vi "Align Image Stacks.vi"(8 "error in (no error)":errorcluster, 10 "Transmitted Light Stack":T1[](array[typedef]), 11 "Reflected Light Stack":T1[](array[typedef])) -> (0 "error out":errorcluster, 3 "Offset":cluster{"dx":i32, "dy":i32})   [LabVIEW 2013]
uses:
  <vilib>/vision/Image Controls.llb/IMAQ Image.ctl
  <vilib>/vision/NI_Vision_Development_Module.lvlib
panel:
  # "The \"Offset\" is the displacement necessary\nto align the reflected light stack with\nthe transmitted light stack. Shift the \nreflected light stack, not the transmitted!"
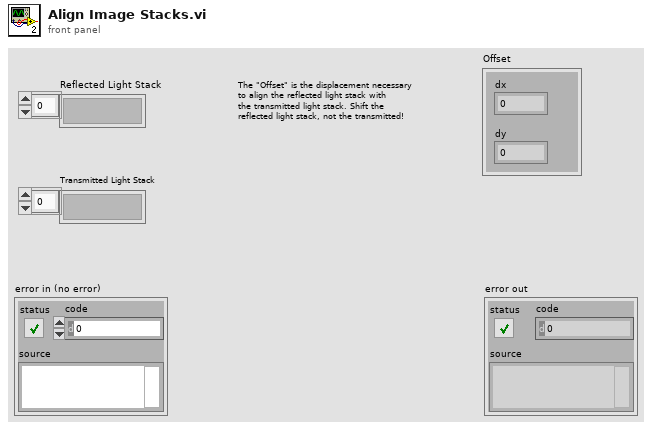
[diagram p1: front panel]
types:
  T1 = typedef "IMAQ Image.ctl" = refnum<image>
  T2 = cluster{"Number of Matches Requested":i32, "Minimum Match Score":sgl, "Angle Ranges":cluster{"Start Angle":sgl, "End Angle":sgl}[]}
  T3 = cluster{"Position":cluster{"X":sgl, "Y":sgl}, "Orientation":dbl, "Major Radius":dbl, "Minor Radius":dbl, "Score":dbl}[]
  T4 = cluster{"Position":cluster{"x":sgl, "y":sgl}, "Angle":sgl, "Scale":sgl, "Score":sgl, "Bounding Box":cluster{"x":sgl, "y":sgl}[]}[]
  T5 = cluster{"Position":cluster{"x":sgl, "y":sgl}, "Angle":sgl, "Scale":sgl, "Score":sgl, "Bounding Box":cluster{"x":sgl, "y":sgl}[]}
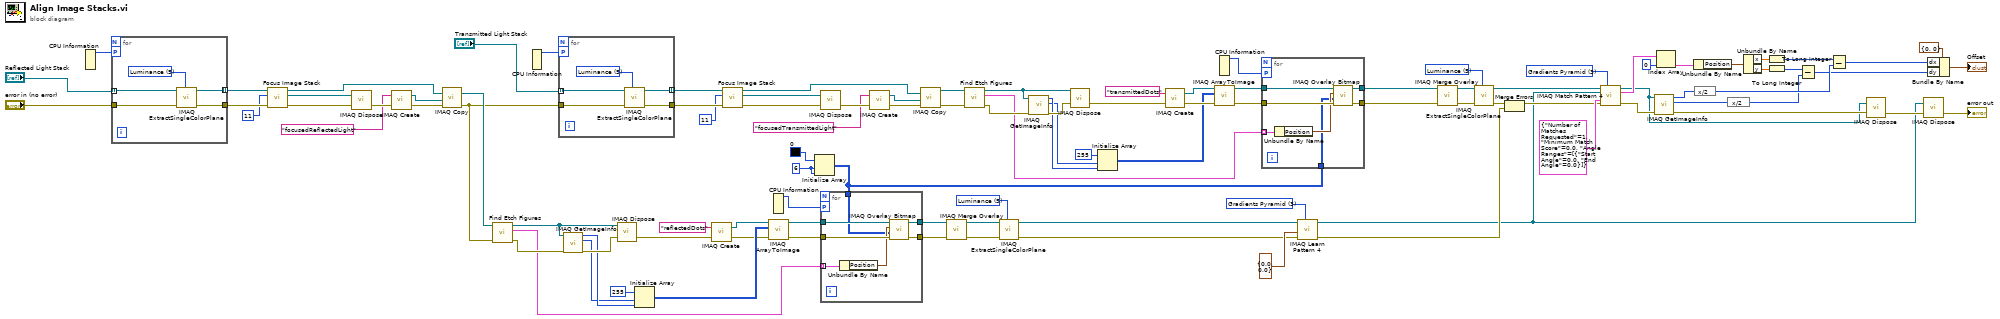
[diagram p0: block diagram]
diagram:
  w4 = 6 ("dimension size")
  w10 = 5 items=["Red", "Green", "Blue", "Hue", "Saturation", "Luminance", "Value", "Intensity"] ("Color Plane")
  w14 = 5 items=["Red", "Green", "Blue", "Hue", "Saturation", "Luminance", "Value", "Intensity"] ("Color Plane")
  w46 = 3 items=["All", "Low Discrepancy Sampling", "Grayscale Value Pyramid", "Gradients Pyramid"] ("Algorithm")
  w47 = 3 items=["All", "Low Discrepancy Sampling", "Grayscale Value Pyramid", "Gradients Pyramid"] ("Algorithm")
  n1 = CPU Information() -> (4:w103:i32)  [unwired: 3 out]
  n2 = for {
    tunnel: "error in (no error)" -> [w109]
    tunnel: "Reflected Light Stack" -> [w108] mode=indexing
    tunnel: [w107] -> w101 mode=indexing
    tunnel: [w106] -> w100
    workers-P: w103 -> [_]
    w105 = 5 items=["Red", "Green", "Blue", "Hue", "Saturation", "Luminance", "Value", "Intensity"] ("Color Plane")
    n3 = call "IMAQ ExtractSingleColorPlane"("Color Plane"=w105, "error in (no error)"=w109, "Image Src"=w108) -> ("error out"=w106:errorcluster, "Image Dst Out"=w107:T1)  [unwired: 7 in]
  }
  n4 = call "Focus Image Stack.vi"("error in (no error)"=w100, "Kernel Size"=11, "Image Stack"=w101) -> ("error out"=w97:errorcluster, "Height Map"=w95:T1, "Focused Image"=w93:T1)  [unwired: 6 in]
  n5 = call "IMAQ Dispose"("Image"=w95, "error in (no error)"=w97) -> ("error out"=w96:errorcluster)  [unwired: 4 in]
  n6 = call "IMAQ Create"("Image Name"="focusedReflectedLight", "error in (no error)"=w96) -> ("New Image"=w92:T1, "error out"=w98:errorcluster)  [unwired: 3 in]
  n7 = call "IMAQ Copy"("error in (no error)"=w98, "Image Dst"=w92, "Image Src"=w93) -> ("error out"=w78:errorcluster, "Image Dst Out"=w79:T1)  [unwired: 3 in]
  n8 = call "Find Etch Figures.vi"("error in"=w78, "Image In"=w79) -> ("error out"=w74:errorcluster, "Etch Figures"=w64:T3, "Image Out"=w73:T1)  [unwired: 7 in]
  n9 = CPU Information() -> (4:w91:i32)  [unwired: 3 out]
  n10 = for {
    tunnel: w78 -> [w114]
    tunnel: "Transmitted Light Stack" -> [w113] mode=indexing
    tunnel: [w112] -> w88 mode=indexing
    tunnel: [w111] -> w89
    workers-P: w91 -> [_]
    w110 = 5 items=["Red", "Green", "Blue", "Hue", "Saturation", "Luminance", "Value", "Intensity"] ("Color Plane")
    n11 = call "IMAQ ExtractSingleColorPlane"("Color Plane"=w110, "error in (no error)"=w114, "Image Src"=w113) -> ("error out"=w111:errorcluster, "Image Dst Out"=w112:T1)  [unwired: 7 in]
  }
  n12 = call "IMAQ GetImageInfo"("error in (no error)"=w74, "Image"=w73) -> ("error out"=w72:errorcluster, "Y Resolution"=w7:i32, "X Resolution"=w8:i32)  [unwired: 2 in, 5 out]
  n13 = call "IMAQ Dispose"("Image"=w73, "error in (no error)"=w72) -> ("error out"=w70:errorcluster)  [unwired: 4 in]
  n14 = Initialize Array(u8 255, w7, w8) -> (w71:u8[][])
  n15 = call "IMAQ Create"("Image Name"="reflectedDots", "error in (no error)"=w70) -> ("New Image"=w68:T1, "error out"=w69:errorcluster)  [unwired: 3 in]
  n16 = call "Focus Image Stack.vi"("error in (no error)"=w89, "Kernel Size"=11, "Image Stack"=w88) -> ("error out"=w86:errorcluster, "Height Map"=w85:T1, "Focused Image"=w80:T1)  [unwired: 6 in]
  n17 = CPU Information() -> (4:w49:i32)  [unwired: 3 out]
  n18 = call "IMAQ ArrayToImage"("error in (no error)"=w69, "Image Pixels (U8)"=w71, "Image"=w68) -> ("error out"=w66:errorcluster, "Image Out"=w65:T1)  [unwired: 7 in]
  n19 = Initialize Array(u32 0, w4, w4) -> (w5:u32[][])
  n20 = for {
    tunnel: w66 -> [w119]
    tunnel: w65 -> [w120]
    tunnel: w64 -> [w121] mode=indexing
    tunnel: [w118] -> w38
    tunnel: [w117] -> w39
    workers-P: w49 -> [_]
    tunnel: w5 -> [w115]
    n21 = Unbundle By Name(w121) -> ("Position"=w116:cluster{"X":sgl, "Y":sgl})
    n22 = call "IMAQ Overlay Bitmap"("error in (no error)"=w119, "Bitmap"=w115, "Top Left Point"=w116, "Image"=w120) -> ("error out"=w117:errorcluster, "Image Out"=w118:T1)  [unwired: 6 in]
  }
  n23 = call "IMAQ Dispose"("Image"=w85, "error in (no error)"=w86) -> ("error out"=w82:errorcluster)  [unwired: 4 in]
  n24 = call "IMAQ Create"("Image Name"="focusedTransmittedLight", "error in (no error)"=w82) -> ("New Image"=w83:T1, "error out"=w84:errorcluster)  [unwired: 3 in]
  n25 = call "IMAQ Copy"("error in (no error)"=w84, "Image Dst"=w83, "Image Src"=w80) -> ("error out"=w76:errorcluster, "Image Dst Out"=w77:T1)  [unwired: 3 in]
  n26 = call "IMAQ Merge Overlay"("error in (no error)"=w39, "Image Src"=w38) -> ("error out"=w15:errorcluster, "Image Dst Out"=w16:T1)  [unwired: 8 in]
  n27 = call "Find Etch Figures.vi"("error in"=w76, "Image In"=w77) -> ("error out"=w63:errorcluster, "Etch Figures"=w50:T3, "Image Out"=w61:T1)  [unwired: 7 in]
  n28 = call "IMAQ ExtractSingleColorPlane"("Color Plane"=w14, "error in (no error)"=w15, "Image Src"=w16) -> ("error out"=w6:errorcluster, "Image Dst Out"=w2:T1)  [unwired: 7 in]
  n29 = call "IMAQ GetImageInfo"("error in (no error)"=w63, "Image"=w61) -> ("error out"=w62:errorcluster, "Y Resolution"=w58:i32, "X Resolution"=w59:i32)  [unwired: 2 in, 5 out]
  n30 = call "IMAQ Dispose"("Image"=w61, "error in (no error)"=w62) -> ("error out"=w56:errorcluster)  [unwired: 4 in]
  n31 = Initialize Array(u8 255, w58, w59) -> (w53:u8[][])
  n32 = call "IMAQ Create"("Image Name"="transmittedDots", "error in (no error)"=w56) -> ("New Image"=w54:T1, "error out"=w55:errorcluster)  [unwired: 3 in]
  n33 = CPU Information() -> (4:w48:i32)  [unwired: 3 out]
  n34 = call "IMAQ ArrayToImage"("error in (no error)"=w55, "Image Pixels (U8)"=w53, "Image"=w54) -> ("error out"=w51:errorcluster, "Image Out"=w52:T1)  [unwired: 7 in]
  n35 = for {
    tunnel: w51 -> [w124]
    tunnel: w52 -> [w125]
    tunnel: w50 -> [w128] mode=indexing
    tunnel: [w127] -> w36
    tunnel: [w126] -> w37
    workers-P: w48 -> [_]
    tunnel: w5 -> [w122]
    n36 = Unbundle By Name(w128) -> ("Position"=w123:cluster{"X":sgl, "Y":sgl})
    n37 = call "IMAQ Overlay Bitmap"("error in (no error)"=w124, "Bitmap"=w122, "Top Left Point"=w123, "Image"=w125) -> ("error out"=w126:errorcluster, "Image Out"=w127:T1)  [unwired: 6 in]
  }
  n38 = call "IMAQ Learn Pattern 4"("Algorithm"=w47, "error in (no error)"=w6, "Angle Range"=cluster{"Start Angle":sgl, "End Angle":sgl} {"Start Angle"=0.0, "End Angle"=0.0}, "Image"=w2) -> ("error out"=w44:errorcluster, "Template Image Out"=w18:T1)  [unwired: 5 in, 1 out]
  n39 = call "IMAQ Merge Overlay"("error in (no error)"=w37, "Image Src"=w36) -> ("error out"=w12:errorcluster, "Image Dst Out"=w13:T1)  [unwired: 8 in]
  n40 = call "IMAQ ExtractSingleColorPlane"("Color Plane"=w10, "error in (no error)"=w12, "Image Src"=w13) -> ("error out"=w11:errorcluster, "Image Dst Out"=w1:T1)  [unwired: 7 in]
  n41 = Merge Errors(w11, w44) -> (w43:errorcluster)
  n42 = call "IMAQ Match Pattern 4"("Image"=w1, "Algorithm"=w46, "Template Image"=w18, "Parameters"=T2 {"Number of Matches Requested"=1, "Minimum Match Score"=0.0, "Angle Ranges"=[{"Start Angle"=0.0, "End Angle"=0.0}]}, "error in (no error)"=w43) -> ("Image (duplicate)"=w19:T1, "Matches (pixel)"=w42:T4, "error out"=w35:errorcluster)  [unwired: 6 in, 2 out]
  n43 = call "IMAQ GetImageInfo"("error in (no error)"=w35, "Image"=w19) -> ("error out"=w21:errorcluster, "Y Resolution"=w28:i32, "X Resolution"=w31:i32)  [unwired: 2 in, 5 out]
  n44 = Index Array(array=w42, index=0) -> (element=w40:T5)
  n45 = Unbundle By Name(w40) -> ("Position"=w34:cluster{"x":sgl, "y":sgl})
  n46 = expression code="x/2"(w31) -> (w27:i32)
  n47 = expression code="x/2"(w28) -> (w26:i32)
  n48 = Unbundle By Name(w34) -> ("x"=w33:sgl, "y"=w32:sgl)
  n49 = To Long Integer(number=w33) -> (32bit integer=w30:i32)
  n50 = To Long Integer(number=w32) -> (32bit integer=w29:i32)
  n51 = Subtract(x=w29, y=w26) -> (x-y=w23:i32)
  n52 = Subtract(x=w30, y=w27) -> (x-y=w24:i32)
  n53 = call "IMAQ Dispose"("Image"=w19, "error in (no error)"=w21) -> ("error out"=w20:errorcluster)  [unwired: 4 in]
  n54 = call "IMAQ Dispose"("Image"=w18, "error in (no error)"=w20) -> ("error out"=→"error out":errorcluster)  [unwired: 4 in]
  n55 = Bundle By Name(cluster=cluster{"dx":i32, "dy":i32} {"dx"=0, "dy"=0} ("Offset"), "dx"=w24, "dy"=w23) -> (→"Offset":cluster{"dx":i32, "dy":i32})
